vi "enable.vi"(8 "error in (no error)":errorcluster, 9 "Parameters":T1, 10 "Model in":refnum<class "Model.lvclass">, 11 "DisabledState in":refnum<class "DisabledState.lvclass">) -> (0 "error out":errorcluster, 2 "Model out":refnum<class "Model.lvclass">, 3 "DisabledState out":refnum<class "DisabledState.lvclass">)   [LabVIEW 2016, in "DisabledState.lvclass"]
uses:
  DisabledState.lvclass
  Model/Model.lvclass
  DataTypes/Topics/CommandEnable.ctl
  DataTypes/Topics/Parts/CommandId.ctl
  DataTypes/Topics/Parts/DetailedStates.ctl
  DataTypes/General/ILCModes.ctl
  DataTypes/Topics/M1M3SupportTopics.lvlib
  DataTypes/General/M1M3SupportGeneral.lvlib
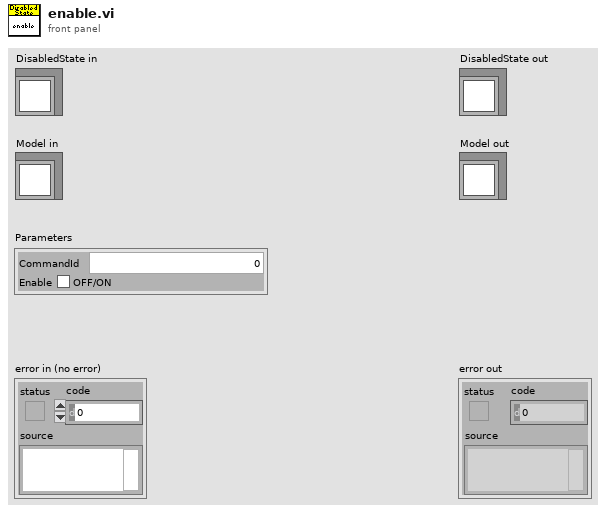
[diagram p1: front panel]
types:
  T1 = typedef "M1M3SupportTopics.lvlib/CommandEnable.ctl" = cluster{"CommandId":T2, "Enable":bool}
  T2 = typedef "M1M3SupportTopics.lvlib/CommandId.ctl" = i32
  T3 = typedef "M1M3SupportTopics.lvlib/DetailedStates.ctl" = enum16{"OfflineState", "InitialState", "StandbyState", "DisabledState", "ParkedState", "FaultState", "ParkedMaintenanceState", "ActiveMaintenanceState"}
  T4 = typedef "M1M3SupportGeneral.lvlib/ILCModes.ctl" = u16
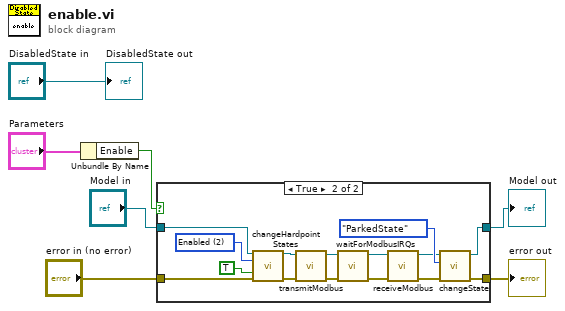
[diagram p0: block diagram]
diagram:
  n1 = Unbundle By Name("Parameters") -> ("Enable"=w1:bool)
  n2 = case shown="True" w1 {
    tunnel: "Model in" -> [w9 w20]
    tunnel: [w9 w23] -> w6
    tunnel: "error in (no error)" -> [w8 w19]
    tunnel: [w8 w22] -> w4
    frame False {
    }
    frame True {
      w10 = T4 2 items=["Standby"=0, "Disabled"=1, "Enabled"=2, "FirmwareUpdate"=3, "Fault"=4, "Status"=65535] ("ILCModes")
      n3 = call "changeHardpointStates.vi"("Model in"=w20, "Mode"=w10, "TriggerIRQ"=TRUE, "error in (no error)"=w19) -> ("Model out"=w18:refnum<class "Model.lvclass">, "error out"=w14:errorcluster)  [unwired: 10 in]
      n4 = call "transmitModbus.vi"("error in (no error)"=w14, "Model in"=w18) -> ("error out"=w13:errorcluster, "Model out"=w17:refnum<class "Model.lvclass">)  [unwired: 8 in]
      n5 = call "waitForModbusIRQs.vi"("error in (no error)"=w13, "Model in"=w17) -> ("error out"=w12:errorcluster, "Model out"=w16:refnum<class "Model.lvclass">)  [unwired: 8 in]
      n6 = call "receiveModbus.vi"("error in (no error)"=w12, "Model in"=w16) -> ("error out"=w11:errorcluster, "Model out"=w15:refnum<class "Model.lvclass">)  [unwired: 8 in]
      n7 = call "changeState.vi"("error in (no error)"=w11, "DetailedStates"=DetailedStates."ParkedState", "Model in"=w15) -> ("error out"=w22:errorcluster, "Model out"=w23:refnum<class "Model.lvclass">)  [unwired: 7 in]
    }
  }
  "error out" <- w4
  "Model out" <- w6
  "DisabledState out" <- "DisabledState in"
